vi "Review.vi"() -> ()   [LabVIEW 2015]
uses:
  oskar_tools/seq_line.ctl
  <vilib>/Analysis/polynomials.llb/Unique Numbers and Multiplicity (DBL).vi
  <vilib>/Analysis/NI_AALPro.lvlib
  oskar_tools/oskar_tools.lvlib
  <vilib>/Analysis/NI_AALBase.lvlib
panel:
  in  "Refresh Button":bool
  out "min":dbl=20.0
  out "max":dbl=101.0
  out "Number":i32=30
  out "Unique":i32=10
  out "Step size (average)":dbl=9.0
  in  "VAR":u16(ring)=2 items=["VAR1", "VAR2", "VAR3"]
  in  "Open (*.jsq)":path
  in  "Tab Control":enum32{"Plot", "Hist", "VARS"}(tab)
  out "Waveform Graph":dbl[][](graph)=[[56.0, 56.0, 56.0, 45.0, 45.0, 45.0, 20.0, 20.0, 20.0, 101.0, 101.0, 101.0, 84.0, 84.0, 84.0, 21.0, 21.0, 21.0, 29.0, 29.0, 29.0, 36.0, 36.0, 36.0, 24.0, 24.0, 24.0, 69.0, 69.0, 69.0], [20.0, 20.0, 20.0, 21.0, 21.0, 21.0, 24.0, 24.0, 24.0, 29.0, 29.0, 29.0, 36.0, 36.0, 36.0, 45.0, 45.0, 45.0, 56.0, 56.0, 56.0, 69.0, 69.0, 69.0, 84.0, 84.0, 84.0, 101.0, 101.0, 101.0]]
  out "Histogram Graph":T1(graph)={"X Values"=[24.05, 32.15, 40.25, 48.35, 56.45, 64.55, 72.65, 80.75, 88.85, 96.95], "Histogram: h(x)"=[9, 6, 0, 3, 3, 0, 3, 3, 0, 3]}
  in  "intervals":i32=10
  out "VAR names":string[](array[string])
  out "SEQs":T2[](array[typedef])=[{"VARS"=[["CHAN_A", "20"], ["CHAN_B", "14"], ["CHAN_C", "56.00"]], "Comment"=""}, {"VARS"=[["CHAN_A", "10"], ["CHAN_B", "14"], ["CHAN_C", "56.00"]], "Comment"=""}, {"VARS"=[["CHAN_A", "0"], ["CHAN_B", "14"], ["CHAN_C", "56.00"]], "Comment"=""}, {"VARS"=[["CHAN_A", "20"], ["CHAN_B", "14"], ["CHAN_C", "45.00"]], "Comment"=""}, {"VARS"=[["CHAN_A", "10"], ["CHAN_B", "14"], ["CHAN_C", "45.00"]], "Comment"=""}, {"VARS"=[["CHAN_A", "0"], ["CHAN_B", "14"], ["CHAN_C", "45.00"]], "Comment"=""}, {"VARS"=[["CHAN_A", "20"], ["CHAN_B", "14"], ["CHAN_C", "20.00"]], "Comment"=""}, {"VARS"=[["CHAN_A", "10"], ["CHAN_B", "14"], ["CHAN_C", "20.00"]], "Comment"=""}, {"VARS"=[["CHAN_A", "0"], ["CHAN_B", "14"], ["CHAN_C", "20.00"]], "Comment"=""}, {"VARS"=[["CHAN_A", "20"], ["CHAN_B", "14"], ["CHAN_C", "101.00"]], "Comment"=""}, {"VARS"=[["CHAN_A", "10"], ["CHAN_B", "14"], ["CHAN_C", "101.00"]], "Comment"=""}, {"VARS"=[["CHAN_A", "0"], ["CHAN_B", "14"], ["CHAN_C", "101.00"]], "Comment"=""}, {"VARS"=[["CHAN_A", "20"], ["CHAN_B", "14"], ["CHAN_C", "84.00"]], "Comment"=""}, {"VARS"=[["CHAN_A", "10"], ["CHAN_B", "14"], ["CHAN_C", "84.00"]], "Comment"=""}, {"VARS"=[["CHAN_A", "0"], ["CHAN_B", "14"], ["CHAN_C", "84.00"]], "Comment"=""}, {"VARS"=[["CHAN_A", "20"], ["CHAN_B", "14"], ["CHAN_C", "21.00"]], "Comment"=""}, {"VARS"=[["CHAN_A", "10"], ["CHAN_B", "14"], ["CHAN_C", "21.00"]], "Comment"=""}, {"VARS"=[["CHAN_A", "0"], ["CHAN_B", "14"], ["CHAN_C", "21.00"]], "Comment"=""}, {"VARS"=[["CHAN_A", "20"], ["CHAN_B", "14"], ["CHAN_C", "29.00"]], "Comment"=""}, {"VARS"=[["CHAN_A", "10"], ["CHAN_B", "14"], ["CHAN_C", "29.00"]], "Comment"=""}, {"VARS"=[["CHAN_A", "0"], ["CHAN_B", "14"], ["CHAN_C", "29.00"]], "Comment"=""}, {"VARS"=[["CHAN_A", "20"], ["CHAN_B", "14"], ["CHAN_C", "36.00"]], "Comment"=""}, {"VARS"=[["CHAN_A", "10"], ["CHAN_B", "14"], ["CHAN_C", "36.00"]], "Comment"=""}, {"VARS"=[["CHAN_A", "0"], ["CHAN_B", "14"], ["CHAN_C", "36.00"]], "Comment"=""}, {"VARS"=[["CHAN_A", "20"], ["CHAN_B", "14"], ["CHAN_C", "24.00"]], "Comment"=""}, {"VARS"=[["CHAN_A", "10"], ["CHAN_B", "14"], ["CHAN_C", "24.00"]], "Comment"=""}, {"VARS"=[["CHAN_A", "0"], ["CHAN_B", "14"], ["CHAN_C", "24.00"]], "Comment"=""}, {"VARS"=[["CHAN_A", "20"], ["CHAN_B", "14"], ["CHAN_C", "69.00"]], "Comment"=""}, {"VARS"=[["CHAN_A", "10"], ["CHAN_B", "14"], ["CHAN_C", "69.00"]], "Comment"=""}, {"VARS"=[["CHAN_A", "0"], ["CHAN_B", "14"], ["CHAN_C", "69.00"]], "Comment"=""}]
  in  "stop":bool
  # "Review"
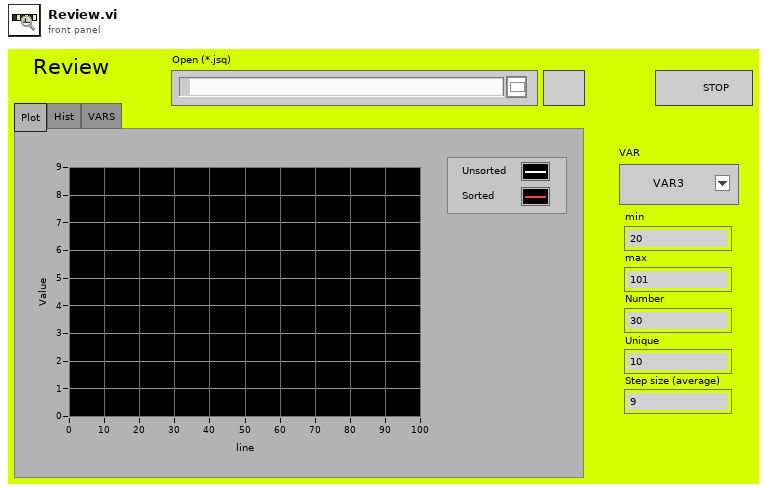
[diagram p1: front panel]
types:
  T1 = cluster{"X Values":dbl[], "Histogram: h(x)":i32[]}
  T2 = typedef "oskar_tools.lvlib/seq_line.ctl" = cluster{"VARS":string[][], "Comment":string}
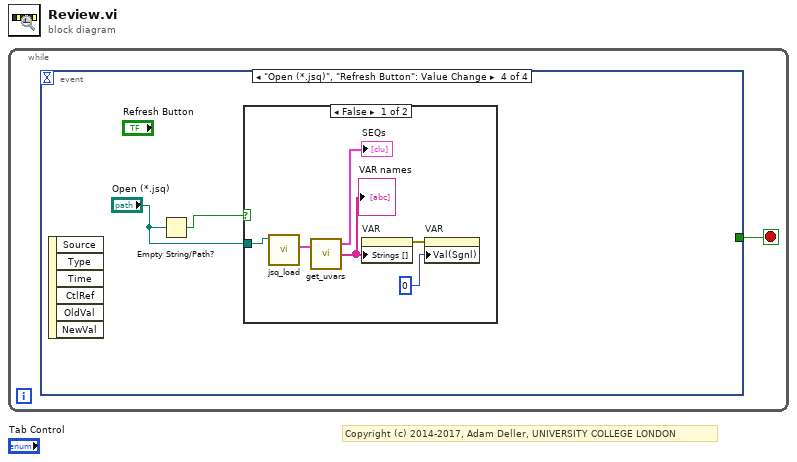
[diagram p0: block diagram]
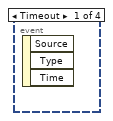
[diagram p2: hidden frame]
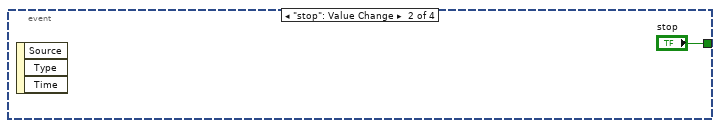
[diagram p3: hidden frame]
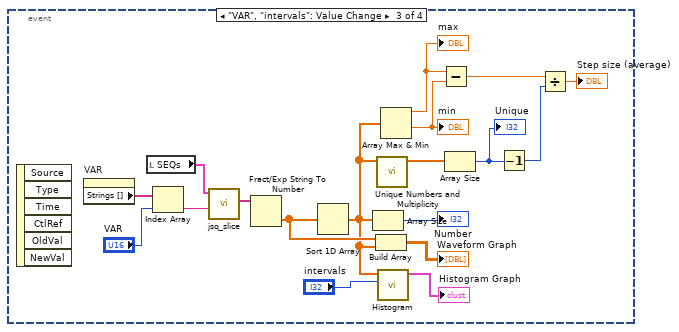
[diagram p4: hidden frame]
diagram:
  # "Copyright (c) 2014-2017, Adam Deller, UNIVERSITY COLLEGE LONDON"
  n1 = while {
    stop <- w1 stop-if-true
    n2 = event shown="[3] \"Open (*.jsq)\", \"Refresh Button\": Value Change" {
      selector: _ -> [_ _ _ _]
      dyn-events: _ -> [_ _ _ _]
      timeout: _ -> [_ _ _ _]
      tunnel: [_ "stop" _ _] -> w1
      event Timeout {
        n3 = event-data() -> ()  [unwired: 1 in, 3 out]
      }
      event "stop": Value Change {
        n4 = event-data() -> ()  [unwired: 1 in, 3 out]
      }
      event "VAR", "intervals": Value Change {
        n5 = event-data() -> ()  [unwired: 1 in, 6 out]
        n6 = property on="VAR" class="Ring (strict)"() -> ("Strings []"=w9:string[])  [unwired: 2 in, 2 out]
        n7 = local read "SEQs"() -> (w10:T2[])
        n8 = Index Array(array=w9, index="VAR") -> (element=w7:string)
        n9 = call "jsq_slice.vi"("VAR"=w7, "SEQs in"=w10) -> ("VALS"=w6:string[])  [unwired: 8 in, 1 out]
        n10 = Fract/Exp String To Number(string=w6) -> (number=w11:dbl[])  [unwired: 3 in, 1 out]
        n11 = Sort 1D Array(array=w11) -> (sorted array=w5:dbl[])
        n12 = Array Size(array=w5) -> (size(s)=→"Number":i32)
        n13 = Build Array(w11, w5) -> (→"Waveform Graph":dbl[][])
        n14 = call-poly <vilib>:"Unique Numbers and Multiplicity.vi"("Numbers"=w5) -> ("Unique Numbers"=w15:dbl[])  [unwired: 8 in, 2 out]
        n15 = call <vilib>:"Histogram.vi"("intervals"="intervals", "X"=w5) -> ("Histogram Graph"=→"Histogram Graph":T1)  [unwired: 6 in, 3 out]
        n16 = Array Max & Min(array=w5) -> (max value=w19:dbl, min value=w14:dbl)  [unwired: 2 out]
        "max" <- w19
        "min" <- w14
        n17 = Subtract(x=w19, y=w14) -> (x-y=w18:dbl)
        n18 = Array Size(array=w15) -> (size(s)=w13:i32)
        "Unique" <- w13
        n19 = Decrement(x=w13) -> (x-1=w12:i32)
        n20 = Divide(x=w18, y=w12) -> (x/y=→"Step size (average)":dbl)
      }
      event "Open (*.jsq)", "Refresh Button": Value Change {
        n21 = event-data() -> ()  [unwired: 1 in, 6 out]
        n22 = Empty String/Path?(string/path="Open (*.jsq)") -> (empty?=w22:bool)
        n23 = case shown="False" w22 {
          tunnel: "Open (*.jsq)" -> [w23 _]
          frame False {
            n24 = call "jsq_load.vi"("Open"=w23) -> ("SEQs"=w26:T2[])  [unwired: 7 in, 3 out]
            n25 = call "get_uvars.vi"("SEQs in"=w26) -> ("SEQs out"=→"SEQs":T2[], "UVARS"=w25:string[])  [unwired: 1 in, 1 out]
            "VAR names" <- w25
            n26 = property on="VAR" class="Ring (strict)"("Strings []"=w25) -> (error out=w27:errorcluster)  [unwired: 2 in, 1 out]
            n27 = property on="VAR" class="Ring (strict)"(error in=w27, "Val(Sgnl)"=u16 0 ("Value (Signaling)")) -> ()  [unwired: 1 in, 2 out]
          }
          frame True {
          }
        }
      }
    }
  }
